vi "Shoot Straight.vi"(8 "error in (no error)":errorcluster, 10 "RPM":dbl) -> (0 "error out":errorcluster)   [LabVIEW 2017]
uses:
  Public/Documents/Cross The Road Electronics/Phoenix-LabVIEW/Motor Controller/Controls/CTRE_Phoenix_MotorControl_ControlMode.ctl
  <vilib>/Rock Robotics/Network Tables/NT Read Number.vi
  Public/Documents/Cross The Road Electronics/Phoenix-LabVIEW/Motor Controller/Get/CTRE_Phoenix_MotorController_GetSelectedSensorData.vi
panel:
  # "if you get too much noise average them"
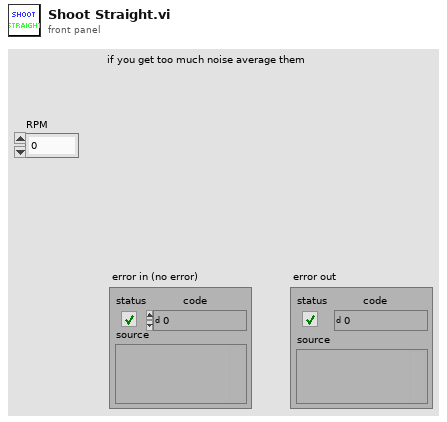
[diagram p1: front panel]
types:
  T1 = typedef "CTRE_Phoenix_MotorControl_ControlMode.ctl" = u16
  T2 = typedef "WPI_MotorControlDeviceRef.ctl" = cluster{"DeviceStatus":errorcluster, "Type":T3, "PWM":cluster{"PWM Channel":T4, "DeadBand":T5}, "CAN":cluster{"Device Number":u8, "SetOutput VI Ref":variant, "GetOutput VI Ref":variant, "Enable VI Ref":variant, "Disable VI Ref":variant, "Data":variant}, "Invert":bool, "DIO PWM":cluster{"PWM \"Enable\" Channel":T4, "DIOChannel":T6, "PWM Rate":dbl}}
  T3 = typedef "WPI_MotorControlType.ctl" = enum16{"PWM", "CAN", "DIO PWM"}
  T4 = typedef "FPGA_DIOPWMChannel.ctl" = enum8{"PWM 0", "PWM 1", "PWM 2", "PWM 3", "PWM 4", "PWM 5", "PWM 6", "PWM 7", "PWM 8", "PWM 9", "PWM MXP 0", "PWM MXP 1", "PWM MXP 2", "PWM MXP 3", "PWM MXP 4", "PWM MXP 5", "PWM MXP 6", "PWM MXP 7", "PWM MXP 8", "PWM MXP 9", "Invalid"}
  T5 = typedef "WPI_PWMDeadband.ctl" = cluster{"Name":string, "maxPositivePwm":i32, "minPositivePwm":i32, "centerPwm":i32, "maxNegativePwm":i32, "minNegativePwm":i32, "angularRange":u16}
  T6 = typedef "FPGA_DIOChannel.ctl" = enum8{"DIO 0", "DIO 1", "DIO 2", "DIO 3", "DIO 4", "DIO 5", "DIO 6", "DIO 7", "DIO 8", "DIO 9", "DIO MXP 0", "DIO MXP 1", "DIO MXP 2", "DIO MXP 3", "DIO MXP 4", "DIO MXP 5", "DIO MXP 6", "DIO MXP 7", "DIO MXP 8", "DIO MXP 9", "DIO MXP 10", "DIO MXP 11", "DIO MXP 12", "DIO MXP 13", "DIO MXP 14", "DIO MXP 15", "SPI Port CS1", "SPI Port CS2", "SPI Port CS3", "SPI Port MISO", "SPI Port MOSI", "Invalid"}
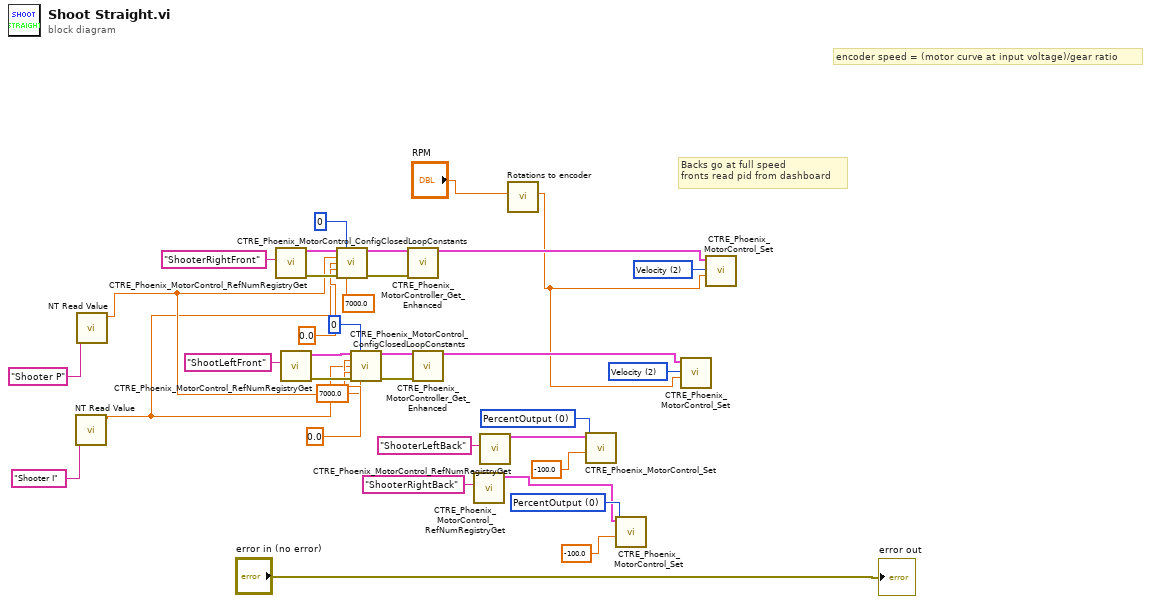
[diagram p0: block diagram]
diagram:
  w3 = T1 0 items=["PercentOutput"=0, "Position"=1, "Velocity"=2, "Current"=3, "Follower"=5, "MotionProfile"=6, "MotionMagic"=7, "MotionMagicArc"=8, "MotionProfileArc"=10, "Disabled"=15] ("Control Mode")
  w6 = T1 0 items=["PercentOutput"=0, "Position"=1, "Velocity"=2, "Current"=3, "Follower"=5, "MotionProfile"=6, "MotionMagic"=7, "MotionMagicArc"=8, "MotionProfileArc"=10, "Disabled"=15] ("Control Mode")
  w31 = T1 2 items=["PercentOutput"=0, "Position"=1, "Velocity"=2, "Current"=3, "Follower"=5, "MotionProfile"=6, "MotionMagic"=7, "MotionMagicArc"=8, "MotionProfileArc"=10, "Disabled"=15] ("Control Mode")
  w32 = T1 2 items=["PercentOutput"=0, "Position"=1, "Velocity"=2, "Current"=3, "Follower"=5, "MotionProfile"=6, "MotionMagic"=7, "MotionMagicArc"=8, "MotionProfileArc"=10, "Disabled"=15] ("Control Mode")
  # "Backs go at full speed\nfronts read pid from dashboard"
  # "encoder speed = (motor curve at input voltage)/gear ratio"
  n1 = call-poly <vilib>:"NT Read Value.vi"("Name"="Shooter I") -> ("Numeric"=w11:dbl)  [unwired: 9 in, 1 out]
  n2 = call-poly <vilib>:"NT Read Value.vi"("Name"="Shooter P") -> ("Numeric"=w13:dbl)  [unwired: 9 in, 1 out]
  n3 = call "CTRE_Phoenix_MotorControl_RefNumRegistryGet.vi"("refnum name"="ShooterRightFront") -> ("error out"=w22:errorcluster, "PhoenixMotorControlDevRef"=w24:T2)  [unwired: 9 in]
  n4 = call "CTRE_Phoenix_MotorControl_RefNumRegistryGet.vi"("refnum name"="ShootLeftFront") -> ("error out"=w19:errorcluster, "PhoenixMotorControlDevRef"=w26:T2)  [unwired: 9 in]
  n5 = call "CTRE_Phoenix_MotorControl_ConfigClosedLoopConstants.vi"("PhoenixMotorControlDevRef"=w24, "slotIdx"=0, "P"=w13, "I"=w11, "D"=0.0 ("P"), "error in (no error)"=w22, "F"=7000.0) -> ("PhoenixMotorControlDevRef"=w23:T2, "error out"=w21:errorcluster)  [unwired: 7 in]
  n6 = call "CTRE_Phoenix_MotorControl_ConfigClosedLoopConstants.vi"("PhoenixMotorControlDevRef"=w26, "slotIdx"=0, "P"=w13, "I"=w11, "D"=0.0 ("P"), "error in (no error)"=w19, "F"=7000.0) -> ("PhoenixMotorControlDevRef"=w25:T2, "error out"=w20:errorcluster)  [unwired: 7 in]
  n7 = call-poly "CTRE_Phoenix_MotorController_Get_Enhanced.vi"("PhoenixMotorControlDevRef"=w23, "error in"=w21) -> ("PhoenixMotorControlDevRef"=w30:T2)  [unwired: 10 in, 3 out]
  n8 = call-poly "CTRE_Phoenix_MotorController_Get_Enhanced.vi"("PhoenixMotorControlDevRef"=w25, "error in"=w20) -> ("PhoenixMotorControlDevRef"=w29:T2)  [unwired: 10 in, 3 out]
  n9 = call "CTRE_Phoenix_MotorControl_RefNumRegistryGet.vi"("refnum name"="ShooterRightBack") -> ("PhoenixMotorControlDevRef"=w2:T2)  [unwired: 9 in, 1 out]
  n10 = call "CTRE_Phoenix_MotorControl_RefNumRegistryGet.vi"("refnum name"="ShooterLeftBack") -> ("PhoenixMotorControlDevRef"=w1:T2)  [unwired: 9 in, 1 out]
  n11 = call "Rotations to encoder.vi"("Rotations"="RPM") -> ("Encoder counts"=w28:dbl)  [unwired: 10 in]
  n12 = call "CTRE_Phoenix_MotorControl_Set.vi"("Output"=-100.0, "Control Mode"=w6, "PhoenixMotorControlDevRef"=w1) -> ()  [unwired: 7 in, 2 out]
  n13 = call "CTRE_Phoenix_MotorControl_Set.vi"("Output"=-100.0, "Control Mode"=w3, "PhoenixMotorControlDevRef"=w2) -> ()  [unwired: 7 in, 2 out]
  n14 = call "CTRE_Phoenix_MotorControl_Set.vi"("Output"=w28, "Control Mode"=w31, "PhoenixMotorControlDevRef"=w29) -> ()  [unwired: 7 in, 2 out]
  n15 = call "CTRE_Phoenix_MotorControl_Set.vi"("Output"=w28, "Control Mode"=w32, "PhoenixMotorControlDevRef"=w30) -> ()  [unwired: 7 in, 2 out]
  "error out" <- "error in (no error)"
